vi "Delta T_v1.vi"(8 "Background":dbl[][](array[numeric]), 9 "FrameData":dbl[][][](array[numeric])) -> (0 "FrameData even":dbl[][][](array[numeric]), 1 "FrameData odd":dbl[][][](array[numeric]), 2 "Delta T":dbl[][](array[numeric]), 3 "Delta T over T":dbl[][](array[numeric]))   [LabVIEW 2020]
uses:
  Random subVIs/Control 1.ctl
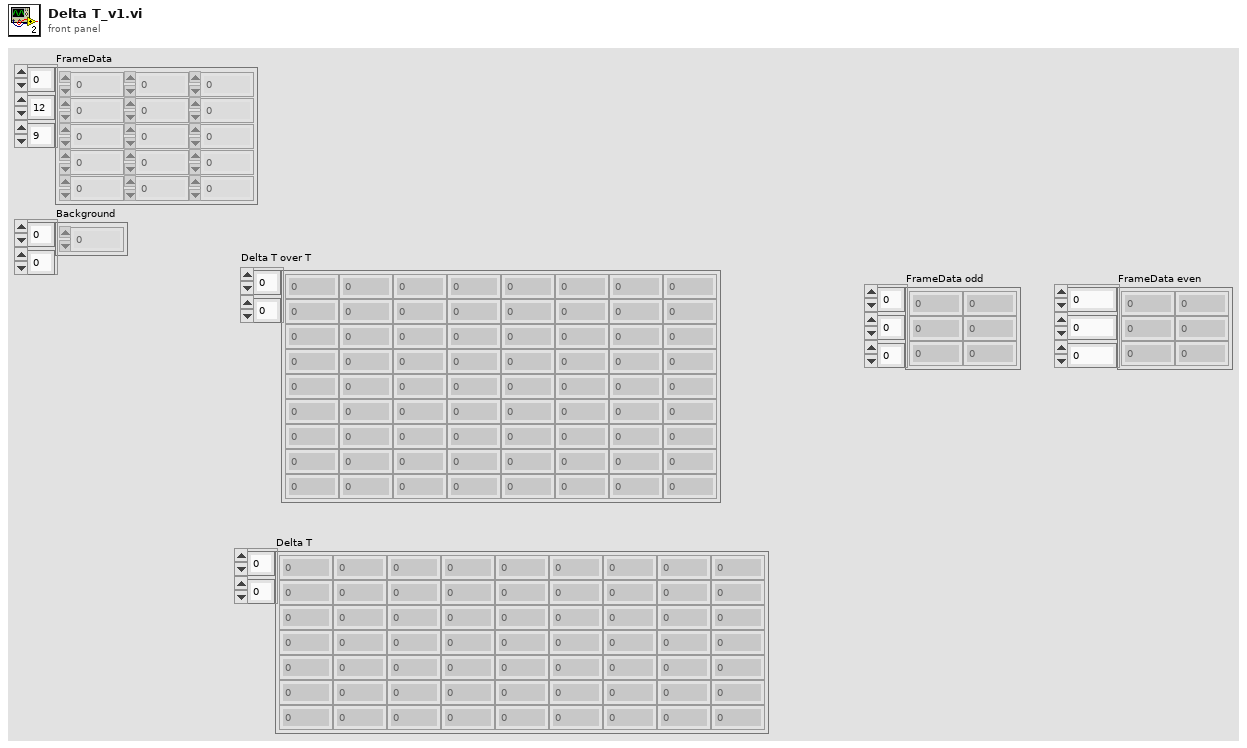
[diagram p1: front panel]
types:
  T1 = typedef "Control 1.ctl" = i32
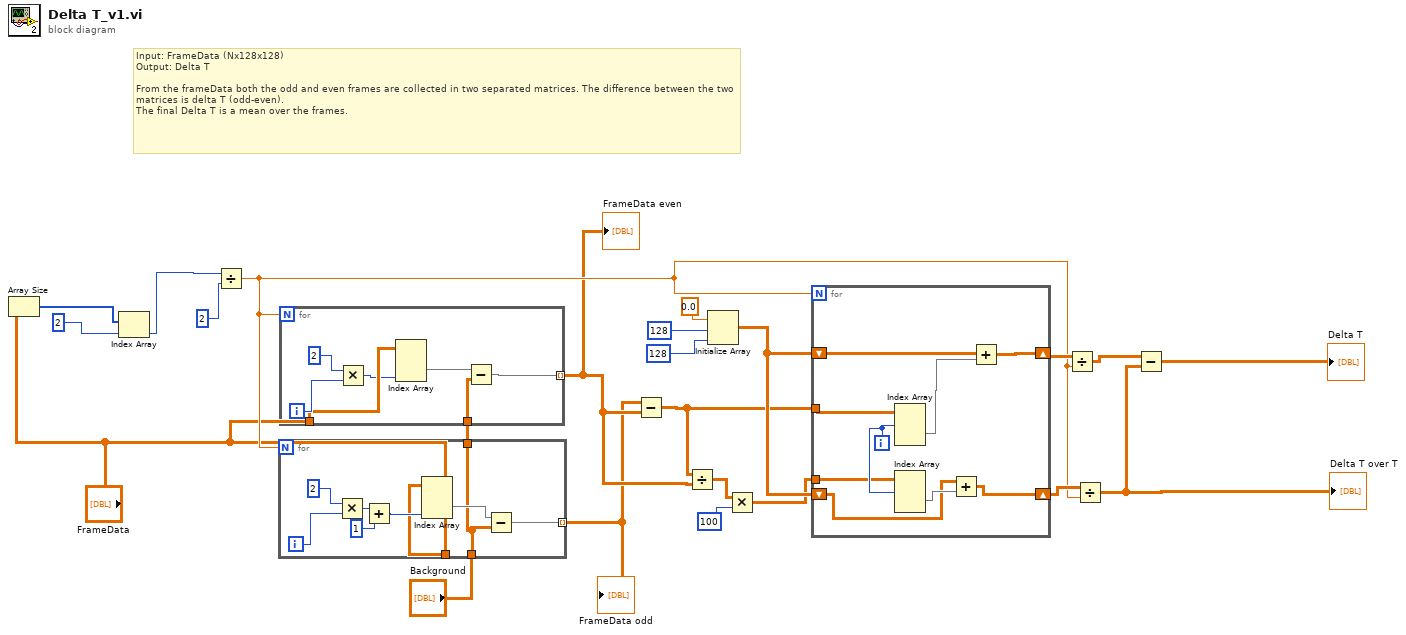
[diagram p0: block diagram]
diagram:
  # "Input: FrameData (Nx128x128)\nOutput: Delta T\n\nFrom the frameData both the odd and even frames are collected in two separated matrices. The difference between the two matrices is delta T (odd-even). \nThe final Delta T is a mean over the frames."
  n1 = Array Size(array="FrameData") -> (size(s)=w17:i32[])
  n2 = Index Array(array=w17, index=2) -> (element=w16:i32)
  n3 = Divide(x=w16, y=T1 2) -> (x/y=w13:dbl)
  n4 = for {
    N: w13 -> [_]
    tunnel: "FrameData" -> [w27]
    tunnel: "Background" -> [w24]
    tunnel: [w25] -> w5 mode=indexing
    tunnel: [w24] -> w4
    i -> [w32]
    n5 = Multiply(x=2, y=w32) -> (x*y=w30:i32)
    n6 = Add(x=w30, y=1) -> (x+y=w28:i32)
    n7 = Index Array(array=w27, index (dim 2)=w28) -> (element=w26:dbl[][])  [unwired: 2 in]
    n8 = Subtract(x=w26, y=w24) -> (x-y=w25:dbl[][])
  }
  "FrameData odd" <- w5
  n9 = for {
    N: w13 -> [_]
    tunnel: [w33] -> w8 mode=indexing
    tunnel: "FrameData" -> [w37]
    tunnel: w4 -> [w34]
    i -> [w39]
    n10 = Multiply(x=2, y=w39) -> (x*y=w36:i32)
    n11 = Index Array(array=w37, index (dim 2)=w36) -> (element=w35:dbl[][])  [unwired: 2 in]
    n12 = Subtract(x=w35, y=w34) -> (x-y=w33:dbl[][])
  }
  "FrameData even" <- w8
  n13 = Subtract(x=w5, y=w8) -> (x-y=w9:dbl[][][])
  n14 = Divide(x=w9, y=w8) -> (x/y=w3:dbl[][][])
  n15 = Initialize Array(0.0 ("element"), 128 ("dimension size"), 128 ("dimension size")) -> (w15:dbl[][])
  n16 = Multiply(x=w3, y=100) -> (x*y=w2:dbl[][][])
  n17 = for {
    N: w13 -> [_]
    tunnel: w9 -> [w48]
    shift-right: [w46] -> w19
    shift-left: w15 -> [w41]
    shift-right: [w43] -> w14
    shift-left: w15 -> [w40]
    tunnel: w2 -> [w42]
    i -> [w45]
    n18 = Index Array(array=w48, index (dim 0)=w45) -> (element=w47:dbl[][])  [unwired: 2 in]
    n19 = Index Array(array=w42, index (dim 0)=w45) -> (element=w44:dbl[][])  [unwired: 2 in]
    n20 = Add(x=w40, y=w44) -> (x+y=w43:dbl[][])
    n21 = Add(x=w41, y=w47) -> (x+y=w46:dbl[][])
  }
  n22 = Divide(x=w19, y=w13) -> (x/y=w11:dbl[][])
  n23 = Divide(x=w14, y=w13) -> (x/y=w7:dbl[][])
  "Delta T over T" <- w7
  n24 = Subtract(x=w11, y=w7) -> (x-y=→"Delta T":dbl[][])
